vi "Init_Time_Synch.vi"(8 "Error in":errorcluster, 11 "Timeout [ms]":i32=3000) -> (0 "Error out":errorcluster, 1 "Synch found?":bool, 2 "Synch Monitor":string[][](table), 3 "Synch Out":refnum<k15>)   [LabVIEW 2021]
uses:
  <instrlib>/niSync/niSync.llb/niSync Initialize (Default).vi
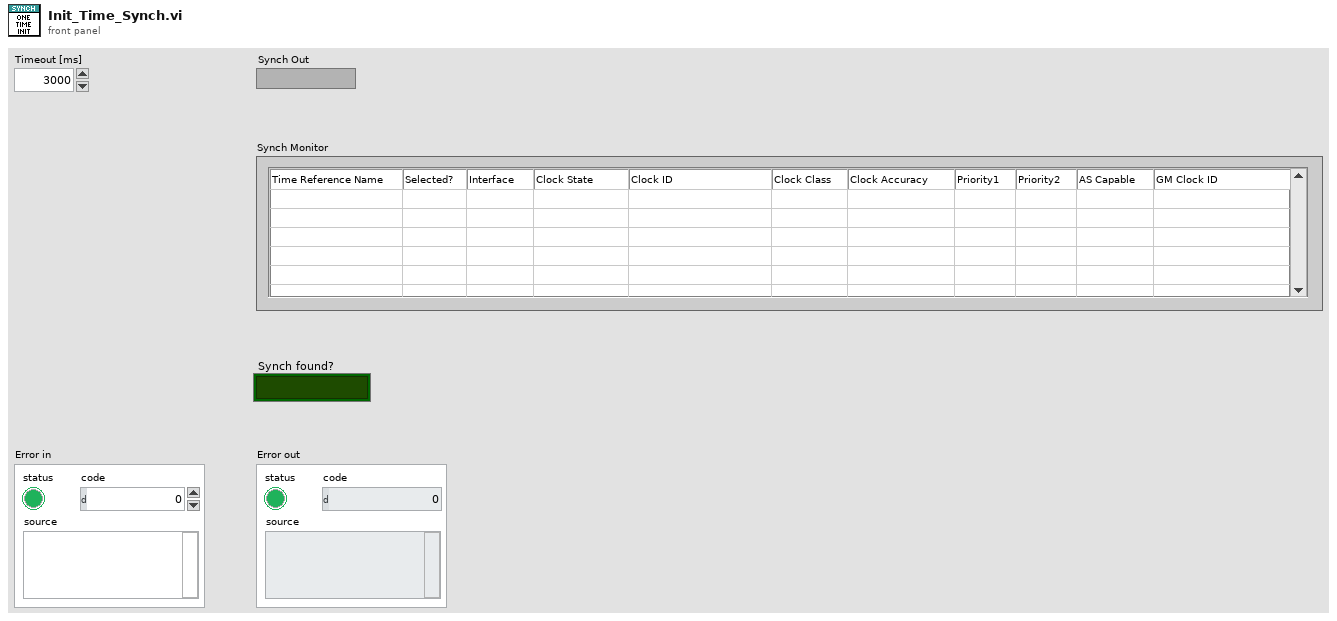
[diagram p1: front panel]
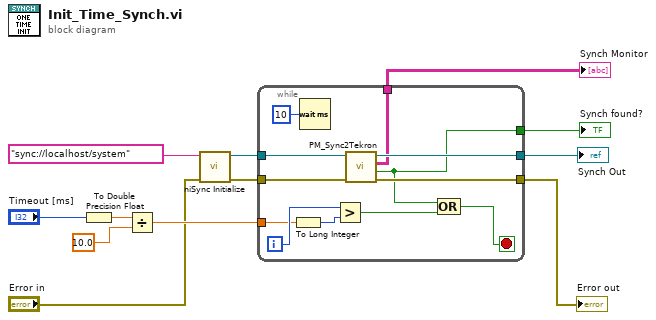
[diagram p0: block diagram]
diagram:
  n1 = To Double Precision Float(number="Timeout [ms]") -> (double precision float=w2:dbl)
  n2 = Divide(x=w2, y=10.0) -> (x/y=w4:dbl)
  n3 = call-poly <instrlib>:"niSync Initialize.vi"("error in (no error)"="Error in", "resource name"=tag "sync://localhost/system") -> ("error out"=w10:errorcluster, "instrument handle out"=w11:refnum<k15>)  [unwired: 8 in]
  n4 = while {
    tunnel: w11 -> [w24]
    tunnel: w10 -> [w18]
    tunnel: [w23] -> w9
    tunnel: w4 -> [w13]
    tunnel: [w17] -> w8
    tunnel: [w16] -> w7
    tunnel: [w15] -> w6
    i -> [w22]
    stop <- w19 stop-if-true
    n5 = To Long Integer(number=w13) -> (32bit integer=w14:i32)
    n6 = Wait (ms)(milliseconds to wait=u32 10) -> ()  [unwired: 1 out]
    n7 = Greater?(x=w22, y=w14) -> (0:w20:bool)
    n8 = call "PM_Sync2Tekron.vi"("instrument handle in"=w24, "error in"=w18) -> ("instrument handle out"=w23:refnum<k15>, "802.1AS Monitor"=w15:string[][], "Synchronized"=w16:bool, "error out"=w17:errorcluster)  [unwired: 5 in]
    n9 = Compound Arithmetic op=OR(w16, w20) -> (w19:bool)
  }
  "Synch Out" <- w9
  "Error out" <- w8
  "Synch found?" <- w7
  "Synch Monitor" <- w6
